vi "SignalGenerator.vi"(0 "Boolean":bool, 1 "Frequency":dbl, 2 "Amplitude":dbl) -> ()   [LabVIEW 2015]
panel:
  out "error out":errorcluster
  in  "error in (no error)":errorcluster
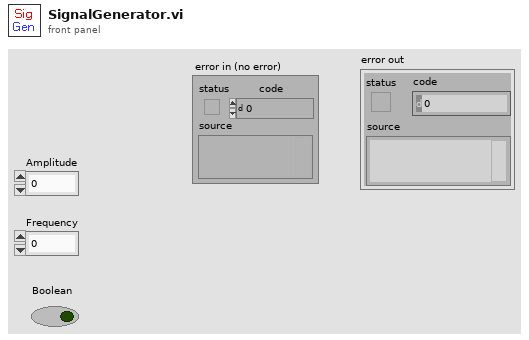
[diagram p1: front panel]
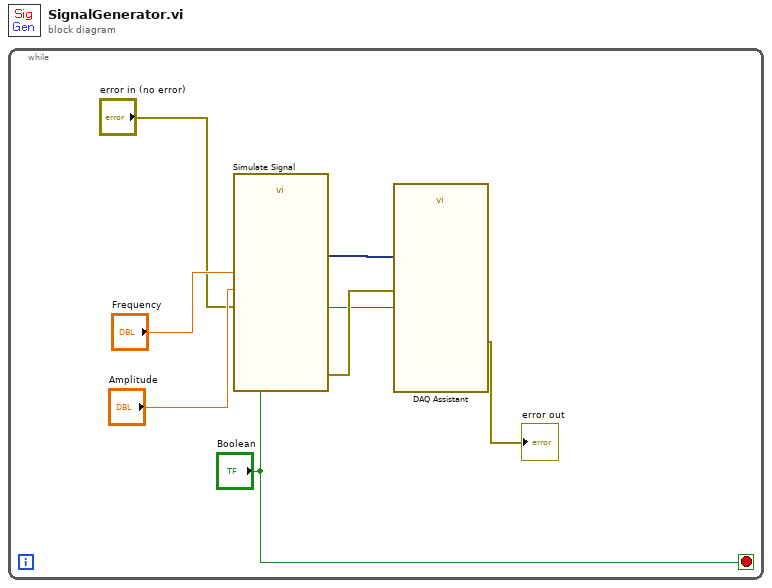
[diagram p0: block diagram]
diagram:
  n1 = while {
    stop <- "Boolean" stop-if-true
    n2 = call "Simulate Signal"("Frequency"="Frequency", "Amplitude"="Amplitude", "error in (no error)"="error in (no error)") -> ("Sine"=w5:dynamicdata, "error out"=w3:errorcluster)  [unwired: 11 in]
    n3 = call "DAQ Assistant"("data"=w5, "error in"=w3, "stop (F)"="Boolean") -> ("error out"=→"error out":errorcluster)  [unwired: 14 in, 2 out]
  }
